vi "Read Y.vi"(8 "error in (no error)":errorcluster, 11 "Data2D in":refnum<class "Data2D.lvclass">) -> (0 "error out":errorcluster, 2 "Y":dbl[](array[numeric]), 3 "Data2D out":refnum<class "Data2D.lvclass">)   [LabVIEW 2018, in "Data2D.lvclass"]
uses:
  Data2D.lvclass
  Data2D.lvclass/Data2D.ctl
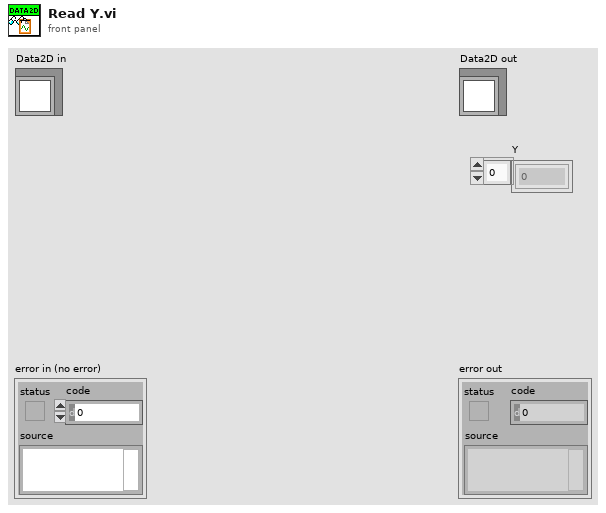
[diagram p1: front panel]
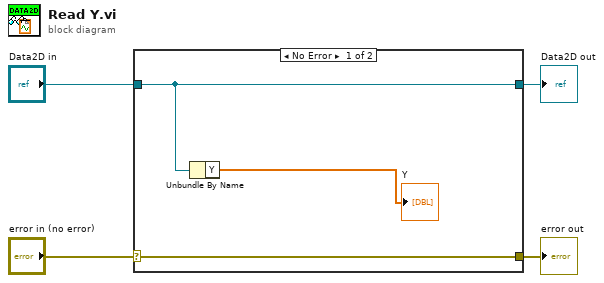
[diagram p0: block diagram]
diagram:
  n1 = case shown="No Error" "error in (no error)" {
    selector: "error in (no error)" -> [w7 w8]
    tunnel: [w7 w8] -> w3
    tunnel: [w6 w9] -> w1
    tunnel: "Data2D in" -> [w6 w9]
    frame No Error {
      n2 = Unbundle By Name(w6) -> ("Y"=→"Y":dbl[])
    }
    frame Error {
    }
  }
  "error out" <- w3
  "Data2D out" <- w1
